vi "gate increment_backup.vi"(10 "Increment":dbl, 11 "Gate Voltage":dbl) -> (2 "Current":string, 3 "Voltage":string)   [LabVIEW 2010]
panel:
  in  "Voltage Safety Limit":dbl
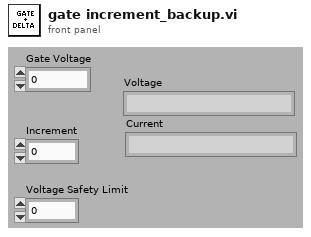
[diagram p1: front panel]
types:
  T1 = enum16{"Set Voltage", "Read Voltage", "Read Setpoint", "Read Current", "Output On", "Output Off"}
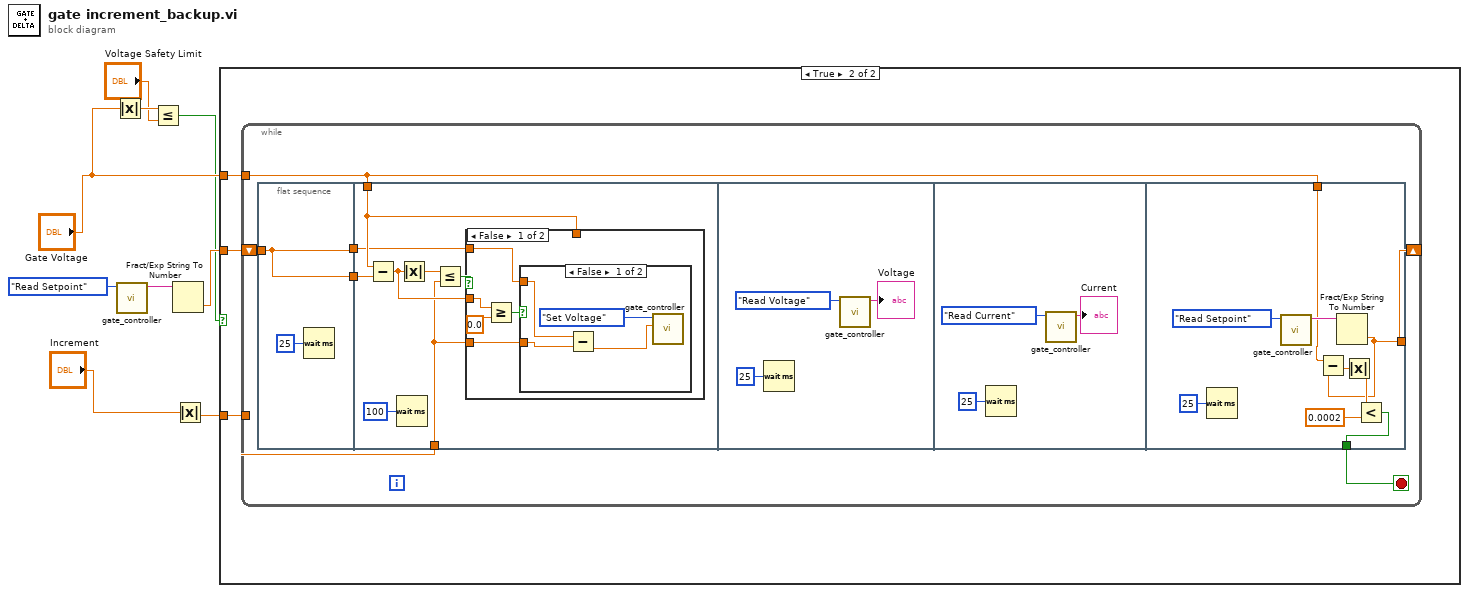
[diagram p0: block diagram]
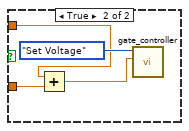
[diagram p3: hidden frame]
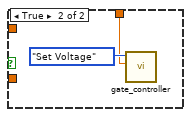
[diagram p4: hidden frame]
diagram:
  n1 = Absolute Value(x="Gate Voltage") -> (abs(x)=w3:dbl)
  n2 = call "gate_controller.vi"("Command"=T1."Read Setpoint") -> ("Response"=w9:string)  [unwired: 10 in]
  n3 = Less Or Equal?(x=w3, y="Voltage Safety Limit") -> (x <= y?=w1:bool)
  n4 = Fract/Exp String To Number(string=w9) -> (number=w7:dbl)  [unwired: 3 in, 1 out]
  n5 = Absolute Value(x="Increment") -> (abs(x)=w6:dbl)
  n6 = case shown="True" w1 {
    tunnel: "Gate Voltage" -> [_ w12]
    tunnel: w7 -> [_ w11]
    tunnel: w6 -> [_ w10]
    frame False {
    }
    frame True {
      n7 = while {
        tunnel: w12 -> [w17]
        tunnel: w10 -> [w18]
        shift-right: [w13] -> _
        shift-left: w11 -> [w14]
        stop <- w16 stop-if-true
        n8 = flat-sequence {
          tunnel: [w20] -> w19
          tunnel: [w20] -> w15
          tunnel: w14 -> [w20]
          tunnel: w17 -> [w26]
          tunnel: w19 -> [w29]
          tunnel: w18 -> [w23]
          tunnel: w15 -> [w22]
          tunnel: w17 -> [w56]
          tunnel: [w52] -> w16
          tunnel: [w51] -> w13
          frame #0 {
            n9 = Wait (ms)(milliseconds to wait=u32 25) -> ()  [unwired: 1 out]
          }
          frame #1 {
            n10 = Subtract(x=w26, y=w29) -> (x-y=w24:dbl)
            n11 = Wait (ms)(milliseconds to wait=u32 100) -> ()  [unwired: 1 out]
            n12 = Absolute Value(x=w24) -> (abs(x)=w28:dbl)
            n13 = Less Or Equal?(x=w28, y=w23) -> (x <= y?=w27:bool)
            n14 = case shown="False" w27 {
              tunnel: w26 -> [_ w43]
              tunnel: w24 -> [w31 _]
              tunnel: w23 -> [w34 _]
              tunnel: w22 -> [w30 _]
              frame False {
                n15 = Greater Or Equal?(x=w31, y=0.0) -> (x >= y?=w33:bool)
                n16 = case shown="False" w33 {
                  tunnel: w34 -> [w36 w41]
                  tunnel: w30 -> [w35 w39]
                  frame False {
                    n17 = Subtract(x=w35, y=w36) -> (x-y=w37:dbl)
                    n18 = call "gate_controller.vi"("Numerical Argument"=w37, "Command"=T1."Set Voltage") -> ()  [unwired: 9 in, 1 out]
                  }
                  frame True {
                    n19 = Add(x=w39, y=w41) -> (x+y=w40:dbl)
                    n20 = call "gate_controller.vi"("Numerical Argument"=w40, "Command"=T1."Set Voltage") -> ()  [unwired: 9 in, 1 out]
                  }
                }
              }
              frame True {
                n21 = call "gate_controller.vi"("Numerical Argument"=w43, "Command"=T1."Set Voltage") -> ()  [unwired: 9 in, 1 out]
              }
            }
          }
          frame #2 {
            n22 = Wait (ms)(milliseconds to wait=u32 25) -> ()  [unwired: 1 out]
            n23 = call "gate_controller.vi"("Command"=T1."Read Voltage") -> ("Response"=→"Voltage":string)  [unwired: 10 in]
          }
          frame #3 {
            n24 = Wait (ms)(milliseconds to wait=u32 25) -> ()  [unwired: 1 out]
            n25 = call "gate_controller.vi"("Command"=T1."Read Current") -> ("Response"=→"Current":string)  [unwired: 10 in]
          }
          frame #4 {
            n26 = Wait (ms)(milliseconds to wait=u32 25) -> ()  [unwired: 1 out]
            n27 = call "gate_controller.vi"("Command"=T1."Read Setpoint") -> ("Response"=w58:string)  [unwired: 10 in]
            n28 = Fract/Exp String To Number(string=w58) -> (number=w51:dbl)  [unwired: 3 in, 1 out]
            n29 = Subtract(x=w56, y=w51) -> (x-y=w55:dbl)
            n30 = Absolute Value(x=w55) -> (abs(x)=w54:dbl)
            n31 = Less?(x=w54, y=0.0002) -> (x < y?=w52:bool)
          }
        }
      }
    }
  }
